vi "LaserCal-Plot Data (PT).vi"(0 "X-Axis":T1, 2 "XY Graph":refnum<vi>, 5 "Parameter":T1, 7 "Fixed Index":i32, 9 "I-O Data in":T2) -> (8 "Array":cluster{"Width":dbl[], dbl[]}[](array[cluster]))   [LabVIEW 2015]
uses:
  Typedefs/LaserCal-Data (PT).ctl
  Typedefs/LaserCal-Plot Param Enum.ctl
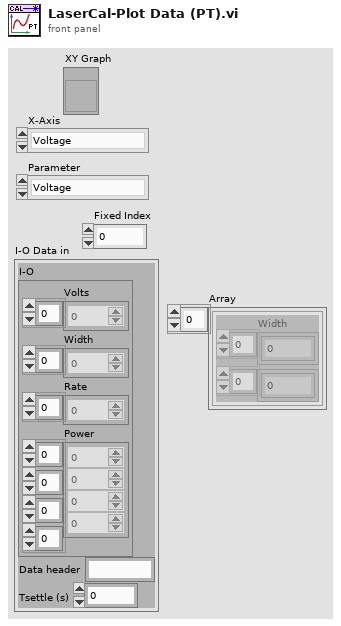
[diagram p1: front panel]
types:
  T1 = typedef "LaserCal-Plot Param Enum.ctl" = enum16{"Voltage", "Width", "Rate"}
  T2 = typedef "LaserCal-Data (PT).ctl" = cluster{"I-O":cluster{"Volts":dbl[], "Width":dbl[], "Rate":dbl[], "Power":dbl[][][][]}, "Data header":string, "Tsettle (s)":dbl}
  T3 = cluster{"Volts":dbl[], "Width":dbl[], "Rate":dbl[], "Power":dbl[][][][]}
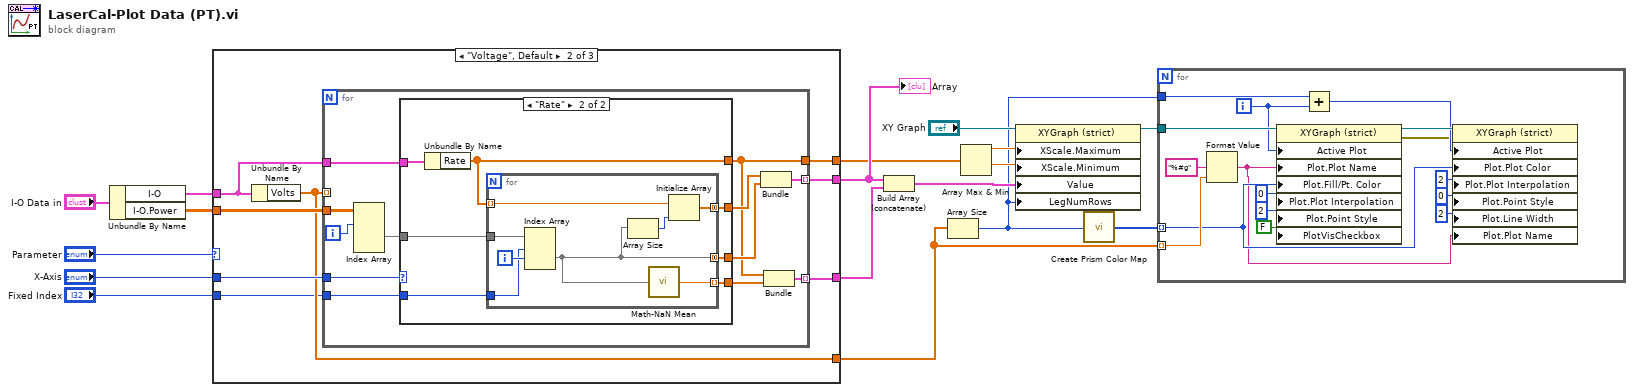
[diagram p0: block diagram]
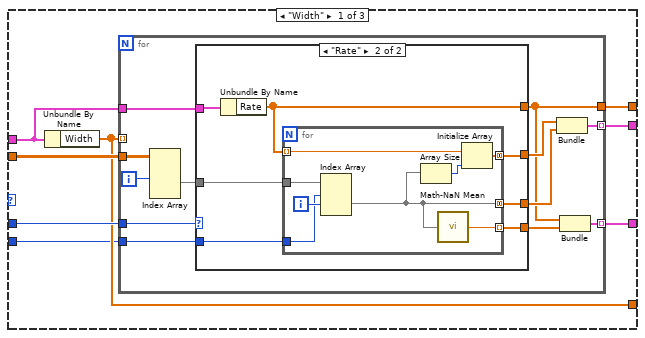
[diagram p2: hidden frame]
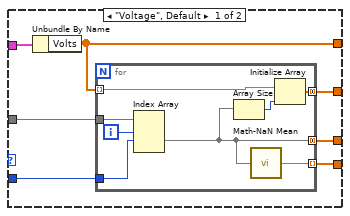
[diagram p3: hidden frame]
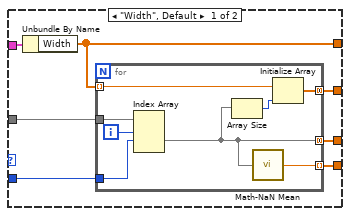
[diagram p4: hidden frame]
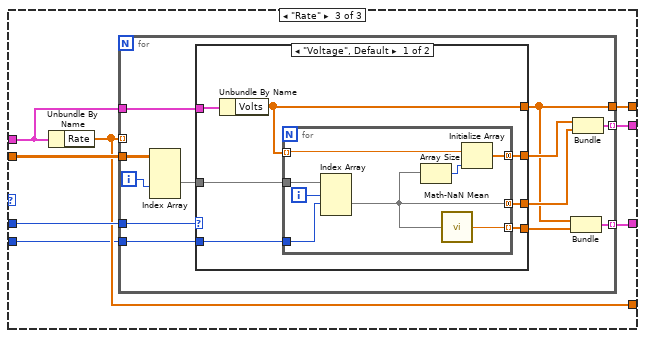
[diagram p5: hidden frame]
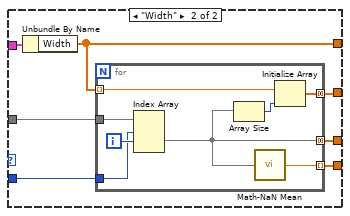
[diagram p6: hidden frame]
diagram:
  n1 = Unbundle By Name("I-O Data in") -> ("I-O"=w14:T3, "I-O.Power"=w17:dbl[][][][])
  n2 = case shown="\"Voltage\", Default" "Parameter" {
    tunnel: w17 -> [w25 w75 w125]
    tunnel: w14 -> [w23 w73 w123]
    tunnel: "X-Axis" -> [w24 w74 w124]
    tunnel: [w22 w72 w122] -> w6
    tunnel: [w21 w71 w121] -> w5
    tunnel: [w20 w70 w120] -> w8
    tunnel: [w19 w69 w119] -> w3
    tunnel: "Fixed Index" -> [w18 w68 w118]
    frame "Width" {
      n3 = Unbundle By Name(w23) -> ("Width"=w21:dbl[])
      n4 = for {
        tunnel: w25 -> [w37]
        tunnel: w21 -> [_] mode=indexing
        tunnel: w24 -> [w35]
        tunnel: w23 -> [w33]
        tunnel: [w28] -> w22
        tunnel: [w31] -> w20 mode=indexing
        tunnel: [w27] -> w19 mode=indexing
        tunnel: w18 -> [w26]
        i -> [w36]
        n5 = Index Array(array=w37, index (dim 1)=w36) -> (element=w34:dbl[][][])  [unwired: 3 in]
        n6 = case shown="\"Rate\"" w35 {
          tunnel: w34 -> [w44 w59]
          tunnel: w33 -> [w43 w58]
          tunnel: [w42 w57] -> w32
          tunnel: [w41 w56] -> w28
          tunnel: [w40 w55] -> w30
          tunnel: [w39 w54] -> w29
          tunnel: w26 -> [w38 w53]
          frame "Voltage", Default {
            n7 = Unbundle By Name(w43) -> ("Volts"=w41:dbl[])
            n8 = for {
              tunnel: w44 -> [w52]
              tunnel: w41 -> [w50] mode=indexing
              tunnel: [w45] -> w42 mode=concatenating
              tunnel: [w48] -> w40 mode=concatenating
              tunnel: [w47] -> w39 mode=indexing
              tunnel: w38 -> [w46]
              i -> [w51]
              n9 = Index Array(array=w52, index (dim 0)=w51, index (dim 1)=w46) -> (element=w45:dbl[])  [unwired: 1 in]
              n10 = Array Size(array=w45) -> (size(s)=w49:i32)
              n11 = call "Math-NaN Mean.vi"("Array"=w45) -> ("NaN Mean"=w47:dbl)
              n12 = Initialize Array(w50, w49) -> (w48:dbl[])
            }
          }
          frame "Rate" {
            n13 = Unbundle By Name(w58) -> ("Rate"=w56:dbl[])
            n14 = for {
              tunnel: w59 -> [w67]
              tunnel: w56 -> [w64] mode=indexing
              tunnel: [w60] -> w57 mode=concatenating
              tunnel: [w63] -> w55 mode=concatenating
              tunnel: [w62] -> w54 mode=indexing
              tunnel: w53 -> [w61]
              i -> [w66]
              n15 = Index Array(array=w67, index (dim 0)=w61, index (dim 1)=w66) -> (element=w60:dbl[])  [unwired: 1 in]
              n16 = Array Size(array=w60) -> (size(s)=w65:i32)
              n17 = call "Math-NaN Mean.vi"("Array"=w60) -> ("NaN Mean"=w62:dbl)
              n18 = Initialize Array(w64, w65) -> (w63:dbl[])
            }
          }
        }
        n19 = Bundle(w30, "Power"=w32) -> (w31:cluster{dbl[], "Power":dbl[]})  [unwired: 1 in]
        n20 = Bundle("Rate"=w28, w29) -> (w27:cluster{"Rate":dbl[], dbl[]})  [unwired: 1 in]
      }
    }
    frame "Voltage", Default {
      n21 = Unbundle By Name(w73) -> ("Volts"=w71:dbl[])
      n22 = for {
        tunnel: w75 -> [w87]
        tunnel: w71 -> [_] mode=indexing
        tunnel: w74 -> [w86]
        tunnel: w73 -> [w84]
        tunnel: [w79] -> w72
        tunnel: [w82] -> w70 mode=indexing
        tunnel: [w77] -> w69 mode=indexing
        tunnel: w68 -> [w76]
        i -> [w81]
        n23 = Index Array(array=w87, index (dim 0)=w81) -> (element=w85:dbl[][][])  [unwired: 3 in]
        n24 = case shown="\"Rate\"" w86 {
          tunnel: w85 -> [w94 w109]
          tunnel: w84 -> [w93 w108]
          tunnel: [w90 w107] -> w83
          tunnel: [w92 w106] -> w79
          tunnel: [w91 w105] -> w80
          tunnel: [w89 w104] -> w78
          tunnel: w76 -> [w88 w103]
          frame "Width", Default {
            n25 = Unbundle By Name(w93) -> ("Width"=w92:dbl[])
            n26 = for {
              tunnel: w94 -> [w102]
              tunnel: w92 -> [w99] mode=indexing
              tunnel: [w98] -> w91 mode=concatenating
              tunnel: [w96] -> w90 mode=concatenating
              tunnel: [w97] -> w89 mode=indexing
              tunnel: w88 -> [w95]
              i -> [w101]
              n27 = Index Array(array=w102, index (dim 0)=w101, index (dim 1)=w95) -> (element=w96:dbl[])  [unwired: 1 in]
              n28 = Array Size(array=w96) -> (size(s)=w100:i32)
              n29 = call "Math-NaN Mean.vi"("Array"=w96) -> ("NaN Mean"=w97:dbl)
              n30 = Initialize Array(w99, w100) -> (w98:dbl[])
            }
          }
          frame "Rate" {
            n31 = Unbundle By Name(w108) -> ("Rate"=w106:dbl[])
            n32 = for {
              tunnel: w109 -> [w117]
              tunnel: w106 -> [w114] mode=indexing
              tunnel: [w110] -> w107 mode=concatenating
              tunnel: [w113] -> w105 mode=concatenating
              tunnel: [w112] -> w104 mode=indexing
              tunnel: w103 -> [w111]
              i -> [w116]
              n33 = Index Array(array=w117, index (dim 0)=w111, index (dim 1)=w116) -> (element=w110:dbl[])  [unwired: 1 in]
              n34 = Array Size(array=w110) -> (size(s)=w115:i32)
              n35 = call "Math-NaN Mean.vi"("Array"=w110) -> ("NaN Mean"=w112:dbl)
              n36 = Initialize Array(w114, w115) -> (w113:dbl[])
            }
          }
        }
        n37 = Bundle(w80, "Power"=w83) -> (w82:cluster{dbl[], "Power":dbl[]})  [unwired: 1 in]
        n38 = Bundle("Rate"=w79, w78) -> (w77:cluster{"Rate":dbl[], dbl[]})  [unwired: 1 in]
      }
    }
    frame "Rate" {
      n39 = Unbundle By Name(w123) -> ("Rate"=w121:dbl[])
      n40 = for {
        tunnel: w125 -> [w137]
        tunnel: w121 -> [_] mode=indexing
        tunnel: w124 -> [w136]
        tunnel: w123 -> [w134]
        tunnel: [w129] -> w122
        tunnel: [w132] -> w120 mode=indexing
        tunnel: [w127] -> w119 mode=indexing
        tunnel: w118 -> [w126]
        i -> [w131]
        n41 = Index Array(array=w137, index (dim 2)=w131) -> (element=w135:dbl[][][])  [unwired: 3 in]
        n42 = case shown="\"Voltage\", Default" w136 {
          tunnel: w135 -> [w144 w159]
          tunnel: w134 -> [w143 w158]
          tunnel: [w142 w157] -> w133
          tunnel: [w141 w156] -> w129
          tunnel: [w140 w155] -> w130
          tunnel: [w139 w154] -> w128
          tunnel: w126 -> [w138 w153]
          frame "Voltage", Default {
            n43 = Unbundle By Name(w143) -> ("Volts"=w141:dbl[])
            n44 = for {
              tunnel: w144 -> [w152]
              tunnel: w141 -> [w149] mode=indexing
              tunnel: [w145] -> w142 mode=concatenating
              tunnel: [w148] -> w140 mode=concatenating
              tunnel: [w147] -> w139 mode=indexing
              tunnel: w138 -> [w146]
              i -> [w151]
              n45 = Index Array(array=w152, index (dim 0)=w151, index (dim 1)=w146) -> (element=w145:dbl[])  [unwired: 1 in]
              n46 = Array Size(array=w145) -> (size(s)=w150:i32)
              n47 = call "Math-NaN Mean.vi"("Array"=w145) -> ("NaN Mean"=w147:dbl)
              n48 = Initialize Array(w149, w150) -> (w148:dbl[])
            }
          }
          frame "Width" {
            n49 = Unbundle By Name(w158) -> ("Width"=w156:dbl[])
            n50 = for {
              tunnel: w159 -> [w167]
              tunnel: w156 -> [w164] mode=indexing
              tunnel: [w160] -> w157 mode=concatenating
              tunnel: [w163] -> w155 mode=concatenating
              tunnel: [w162] -> w154 mode=indexing
              tunnel: w153 -> [w161]
              i -> [w166]
              n51 = Index Array(array=w167, index (dim 0)=w161, index (dim 1)=w166) -> (element=w160:dbl[])  [unwired: 1 in]
              n52 = Array Size(array=w160) -> (size(s)=w165:i32)
              n53 = call "Math-NaN Mean.vi"("Array"=w160) -> ("NaN Mean"=w162:dbl)
              n54 = Initialize Array(w164, w165) -> (w163:dbl[])
            }
          }
        }
        n55 = Bundle("Width"=w129, w128) -> (w127:cluster{"Width":dbl[], dbl[]})  [unwired: 1 in]
        n56 = Bundle(w130, "Power"=w133) -> (w132:cluster{dbl[], "Power":dbl[]})  [unwired: 1 in]
      }
    }
  }
  "Array" <- w8
  n57 = Build Array (concatenate)(w8, w3) -> (w4:cluster{"Width":dbl[], "Power":dbl[]}[])
  n58 = Array Size(array=w5) -> (size(s)=w2:i32)
  n59 = Array Max & Min(array=w6) -> (max value=w11:dbl, min value=w10:dbl)  [unwired: 2 out]
  n60 = property class="XYGraph (strict)"(reference="XY Graph", "XScale.Maximum"=w11, "XScale.Minimum"=w10, "Value"=w4, "LegNumRows"=w2) -> (reference out=w9:refnum<vi>)  [unwired: 1 in, 1 out]
  n61 = call "Create Prism Color Map.vi"("Size"=w2) -> ("Colors"=w7:u32[])
  n62 = for {
    tunnel: w9 -> [w183]
    tunnel: w5 -> [w181] mode=indexing
    tunnel: w7 -> [w173] mode=indexing
    tunnel: w2 -> [w175]
    i -> [w176]
    n63 = Format Value(format string="%#g", value (0)=w181) -> (output string=w168:string)  [unwired: 1 in]
    n64 = property class="XYGraph (strict)"(reference=w183, "Active Plot"=w176, "Plot.Plot Name"=w168, "Plot.Fill/Pt. Color"=w173, "Plot.Plot Interpolation"=u8 0, "Plot.Point Style"=u8 2, "PlotVisCheckbox"=FALSE ("Legend:Plot Visibility Checkbox Visible")) -> (reference out=w177:refnum<vi>, error out=w169:errorcluster)  [unwired: 1 in]
    n65 = Add(x=w175, y=w176) -> (x+y=w174:i32)
    n66 = property class="XYGraph (strict)"(reference=w177, error in=w169, "Active Plot"=w174, "Plot.Plot Color"=w173, "Plot.Plot Interpolation"=u8 2, "Plot.Point Style"=u8 0, "Plot.Line Width"=u8 2, "Plot.Plot Name"=w168) -> ()  [unwired: 2 out]
  }
